vi "Match Regex.vi"(7 "regular expression":string, 8 "error in (no error)":errorcluster, 9 "offset":i32, 11 "String":string) -> (0 "error out":errorcluster, 1 "offset past match":i32, 2 "submatch 1":string, 3 "whole match":string)   [LabVIEW 2015, in "JSON.lvlib"]
uses:
  JSON.lvlib
  <vilib>/regexp/Match Regular Expression.xnode
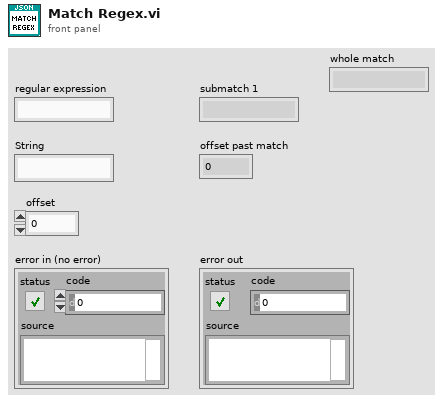
[diagram p1: front panel]
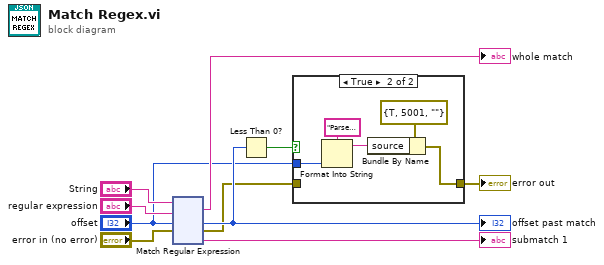
[diagram p0: block diagram]
diagram:
  n1 = xnode "Match Regular Expression"("input string"="String", "regular expression"="regular expression", "offset (0)"="offset", "error in"="error in (no error)") -> ("whole match"=→"whole match":string, "offset past match"=w9:i32, "error out"=w2:errorcluster, "submatch 1"=→"submatch 1":string)  [unwired: 2 in, 2 out]
  "offset past match" <- w9
  n2 = Less Than 0?(x=w9) -> (x < 0?=w4:bool)
  n3 = case shown="True" w4 {
    tunnel: "offset" -> [_ w16]
    tunnel: w2 -> [w11 _]
    tunnel: [w11 w12] -> w1
    frame False {
    }
    frame True {
      n4 = Format Into String(format string="Parse error at %d", w16) -> (resulting string=w13:string)  [unwired: 2 in, 1 out]
      n5 = Bundle By Name(cluster=errorcluster {"status"=TRUE, "code"=5001, "source"=""} ("error constant"), "source"=w13) -> (w12:errorcluster)
    }
  }
  "error out" <- w1
